vi "Sequence Control.vi"() -> ()   [LabVIEW 2014]
uses:
  Support Code/Robot Global Data.vi
panel:
  in  "Sequence":T1(ring)
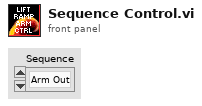
[diagram p1: front panel]
types:
  T1 = enum16{"Arm Out", "All In", "Lift Down", "Ramp Out"}
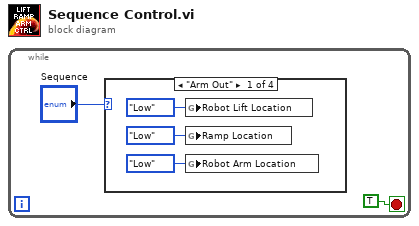
[diagram p0: block diagram]
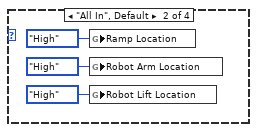
[diagram p2: hidden frame]
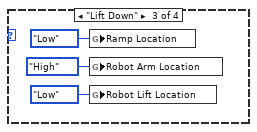
[diagram p3: hidden frame]
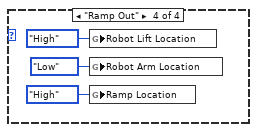
[diagram p4: hidden frame]
diagram:
  n1 = while {
    stop <- TRUE stop-if-true
    n2 = case shown="\"Arm Out\"" "Sequence" {
      frame "Arm Out" {
        n3 = global write "Robot Global Data.vi" "Robot Lift Location"(enum16{"High", "Low"}."Low" ("Robot Lift Location")) -> ()
        n4 = global write "Robot Global Data.vi" "Ramp Location"(enum16{"High", "Low"}."Low" ("Ramp Location")) -> ()
        n5 = global write "Robot Global Data.vi" "Robot Arm Location"(enum16{"High", "Low"}."Low" ("Robot Arm Location")) -> ()
      }
      frame "All In", Default {
        n6 = global write "Robot Global Data.vi" "Ramp Location"(enum16{"High", "Low"}."High" ("Ramp Location")) -> ()
        n7 = global write "Robot Global Data.vi" "Robot Arm Location"(enum16{"High", "Low"}."High" ("Robot Arm Location")) -> ()
        n8 = global write "Robot Global Data.vi" "Robot Lift Location"(enum16{"High", "Low"}."High" ("Robot Lift Location")) -> ()
      }
      frame "Lift Down" {
        n9 = global write "Robot Global Data.vi" "Ramp Location"(enum16{"High", "Low"}."Low" ("Ramp Location")) -> ()
        n10 = global write "Robot Global Data.vi" "Robot Arm Location"(enum16{"High", "Low"}."High" ("Robot Arm Location")) -> ()
        n11 = global write "Robot Global Data.vi" "Robot Lift Location"(enum16{"High", "Low"}."Low" ("Robot Lift Location")) -> ()
      }
      frame "Ramp Out" {
        n12 = global write "Robot Global Data.vi" "Robot Lift Location"(enum16{"High", "Low"}."High" ("Robot Lift Location")) -> ()
        n13 = global write "Robot Global Data.vi" "Robot Arm Location"(enum16{"High", "Low"}."Low" ("Robot Arm Location")) -> ()
        n14 = global write "Robot Global Data.vi" "Ramp Location"(enum16{"High", "Low"}."High" ("Ramp Location")) -> ()
      }
    }
  }
